vi "Exclude Library Items.vi"(7 "Exclude?":bool, 8 "error in (no error)":errorcluster, 11 "BuildSpec in":refnum<vi>) -> (0 "error out":errorcluster, 3 "BuildSpec out":refnum<vi>)   [LabVIEW 2019, in "Project Sync Tools.lvclass"]
uses:
  Project Sync Tools.lvclass
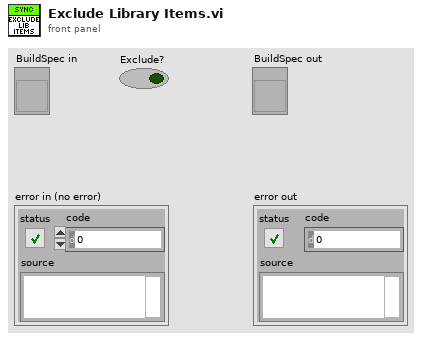
[diagram p1: front panel]
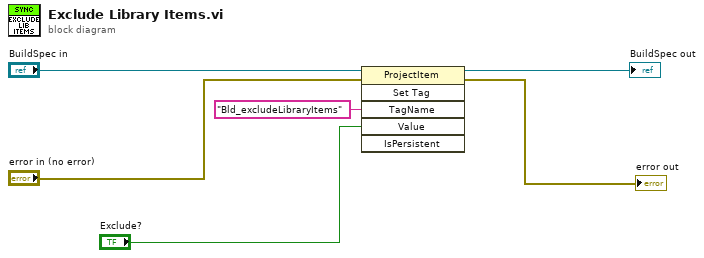
[diagram p0: block diagram]
diagram:
  n1 = invoke class="ProjectItem" method="Set Tag"(reference="BuildSpec in", error in="error in (no error)", "TagName"="Bld_excludeLibraryItems" ("Tag Name"), "Value"="Exclude?") -> (reference out=→"BuildSpec out":refnum<vi>, error out=→"error out":errorcluster)  [unwired: 2 in, 4 out]
